vi "svfa_Compute FFT Subset.vi"(8 "error in (no error)":errorcluster, 9 "frequency range":T1={"start frequency"=20.0, "stop frequency"=20000.0} {"stop frequency" format="%.2f"; "start frequency" format="%.2f"}, 11 "windowed signal":waveform(dbl)={"t0"=timestamp(0 s since 1904-01-01), "dt"=0.0, "Y"=[]}) -> (0 "error out":errorcluster, 3 "FFT spectrum [Vrms]":cluster{"f0":dbl, "df":dbl, "spectrum":cdb[]}={"f0"=0.0, "df"=1.0, "spectrum"=[]} {"spectrum" format="%.2f"; "df" format="%.2f"; "f0" format="%.2f"})   [LabVIEW 2017]
uses:
  <vilib>/Analysis/sml.llb/aal_DZT (real input).vi
  <vilib>/Analysis/NI_AALPro.lvlib
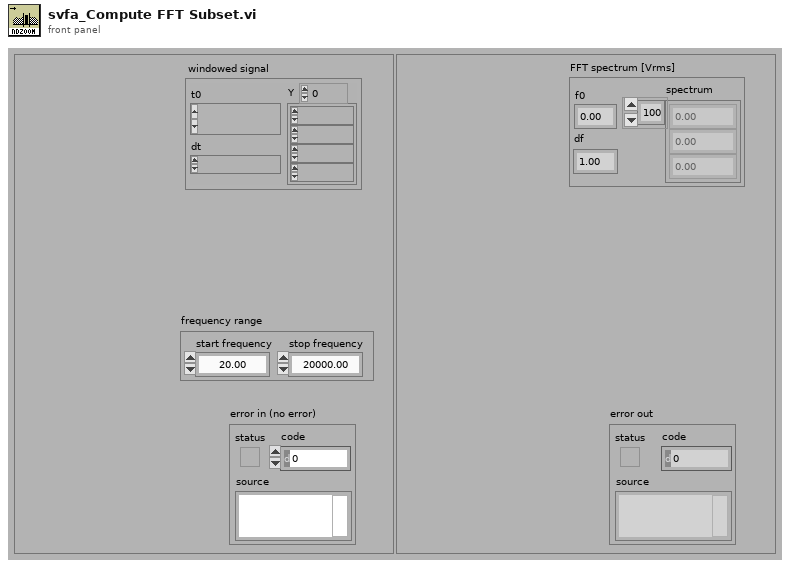
[diagram p1: front panel]
types:
  T1 = cluster{"start frequency":dbl, "stop frequency":dbl}
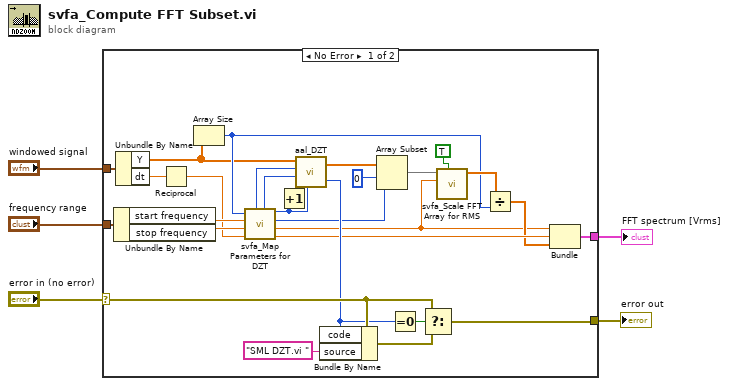
[diagram p0: block diagram]
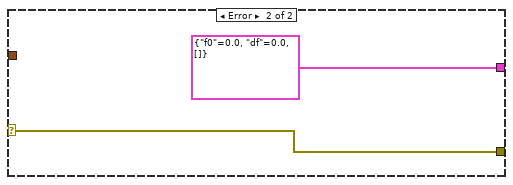
[diagram p2: hidden frame]
diagram:
  n1 = case shown="No Error" "error in (no error)" {
    selector: "error in (no error)" -> [w30 w34]
    tunnel: "windowed signal" -> [w6 _]
    tunnel: [w32 cluster{"f0":dbl, "df":dbl, cdb[]} {"f0"=0.0, "df"=0.0, []}] -> w4
    tunnel: [w33 w34] -> w5
    tunnel: "frequency range" -> [w31 _]
    frame No Error {
      n2 = Unbundle By Name(w31) -> ("start frequency"=w17:dbl, "stop frequency"=w16:dbl)
      n3 = Unbundle By Name ("Get Waveform Components")(w6) -> ("Y"=w8:dbl[], "dt"=w9:dbl)
      n4 = Reciprocal(x=w9) -> (1/x=w7:dbl)
      n5 = Array Size(array=w8) -> (size(s)=w11:i32)
      n6 = call <vilib>:"svfa_Map Parameters for DZT.vi"("fs"=w7, "stop frequency"=w16, "start frequency"=w17, "Block Size"=w11) -> ("df"=w22:dbl, "f0"=w10:dbl, "output length"=w23:i32, "FFT length"=w19:i32, "start index"=w20:i32, "M"=w21:i32)  [unwired: 2 in]
      n7 = Increment(x=w19) -> (x+1=w25:i32)
      n8 = call-poly <vilib>:"aal_DZT.vi"("x"=w8, "M"=w21, "index"=w20, "out_len"=w25, "fft_len"=w19) -> ("Y"=w27:cdb[], "error"=w26:i32)
      n9 = Bundle By Name(cluster=w30, "code"=w26, "source"="SML DZT.vi ") -> (w28:errorcluster)
      n10 = Array Subset(array=w27, index=0 ("32bit integer"), length=w23) -> (w15:cdb[])
      n11 = Equal To 0?(x=w26) -> (x = 0?=w29:bool)
      n12 = Select(t=w30, s=w29, f=w28) -> (s? t:f=w33:errorcluster)
      n13 = call <vilib>:"svfa_Scale FFT Array for RMS.vi"("leave DC bin unscaled (T)"=TRUE ("leave DC bin unscaled"), "f0"=w10, "FFT{X} [EU]"=w15) -> ("FFT {X} [rms]"=w13:cdb[])  [unwired: 8 in]
      n14 = Divide(x=w13, y=w11) -> (x/y=w12:cdb[])
      n15 = Bundle("f0"=w10, "df"=w22, w12) -> (w32:cluster{"f0":dbl, "df":dbl, cdb[]})  [unwired: 1 in]
    }
    frame Error {
    }
  }
  "FFT spectrum [Vrms]" <- w4
  "error out" <- w5
